vi "PFI-28000-Chan-28144_Create.vi"(0 "Model String":string, 11 "error in (no error)":errorcluster) -> (4 "PFI-28000-Chan-28144 out":refnum<class "PFI-28000-Chan-28144.lvclass">, 15 "error out":errorcluster)   [LabVIEW 2017, in "PFI-28000-Chan-28144.lvclass"]
uses:
  PFI-28000-Chan-28144.lvclass
  C:/wc/07143 Precision Filters 28000 Support/Driver/source/Channel/PFI-28000-Channel.lvclass
  28144 Current Channel/PFI-28000-Chan-28144-I.lvclass
  C:/wc/07143 Precision Filters 28000 Support/Driver/source/28144 Channel/PFI-28000-Chan-28144.lvclass
  28144 Voltage Channel/PFI-28000-Chan-28144-V.lvclass
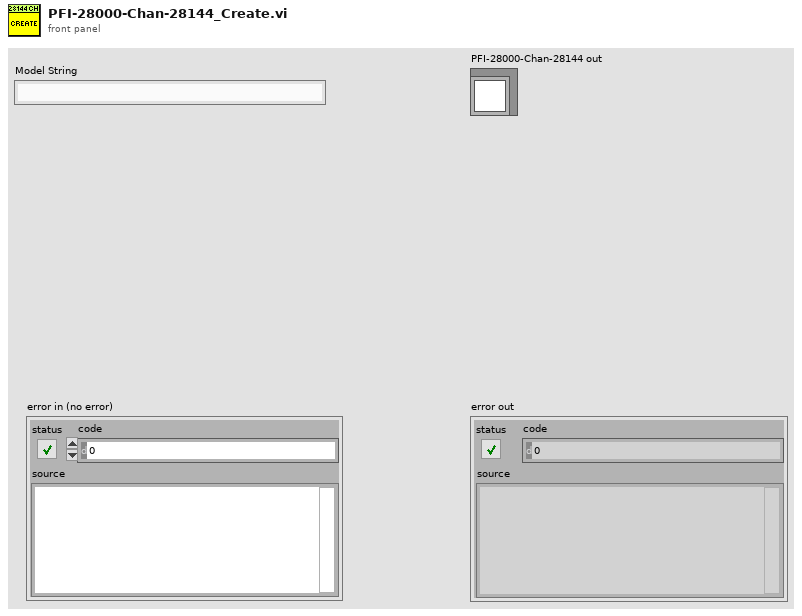
[diagram p1: front panel]
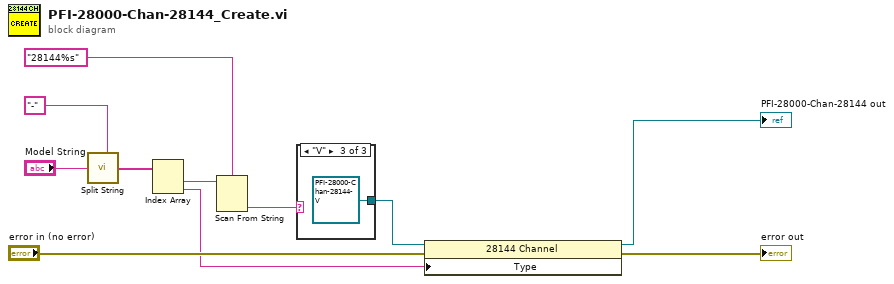
[diagram p0: block diagram]
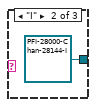
[diagram p3: hidden frame]
diagram:
  n1 = call <vilib>:"Split String.vi"("Split Pattern"="-" ("empty string"), "Input String"="Model String") -> ("Split String"=w9:string[])  [unwired: 5 in]
  n2 = Index Array(array=w9) -> (element #1=w8:string, element #2=w1:string)  [unwired: 2 in]
  n3 = Scan From String(format string="28144%s" ("empty string"), input string=w8) -> (output 1=w6:string)  [unwired: 3 in, 3 out]
  n4 = case shown="\"V\"" w6 {
    tunnel: [_ refnum<class "PFI-28000-Chan-28144-I.lvclass"> refnum ("PFI-28000-Chan-28144-I.lvclass") refnum<class "PFI-28000-Chan-28144-V.lvclass"> refnum ("PFI-28000-Chan-28144-V.lvclass")] -> w5
    frame Default {
    }
    frame "I" {
    }
    frame "V" {
    }
  }
  n5 = property class="28144 Channel"(reference=w5, error in="error in (no error)", "Type"=w1) -> (reference out=→"PFI-28000-Chan-28144 out":refnum<class "PFI-28000-Chan-28144.lvclass">, error out=→"error out":errorcluster)
